vi "GFITS_getInfo.vi"(10 "ID":string, 11 "Database RefNum in":T1) -> (2 "INFO":string[][](array[string]))   [LabVIEW 2016]
uses:
  DBSHAND/private/vis/DatabaseHand_RefNum.ctl
  DBSHAND/private/vis/DatabaseHand_Element_Get(2DArr).vi
panel:
  out "Info received":string[][](table)=[["TIME", "", "time"], ["DATE", "", "data"], ["HRANGLE", "", "hr angle"], ["AZ", "", "az"], ["EI", "", "ei"], ["AIRMASS", "", "airmass"], ["DOME", "", "dome"], ["", "", ""], ["", "", ""]]
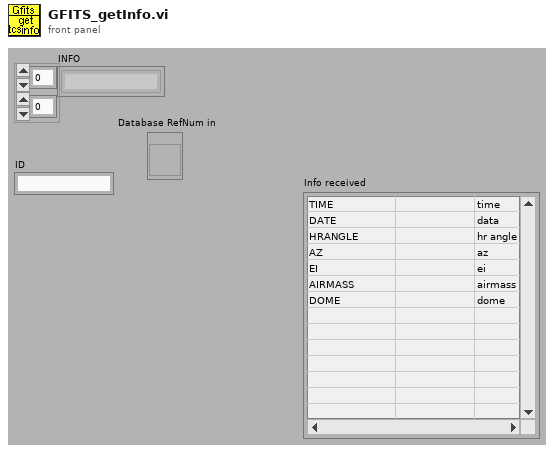
[diagram p1: front panel]
types:
  T1 = typedef "DatabaseHand_RefNum.ctl" = refnum<vi>
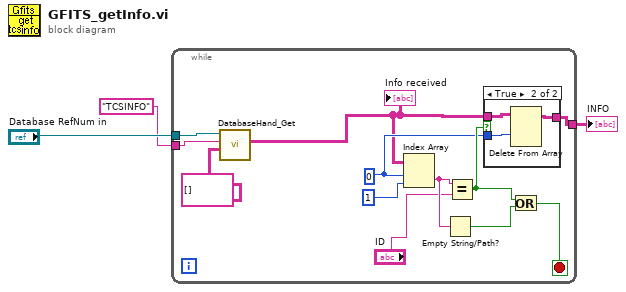
[diagram p0: block diagram]
diagram:
  n1 = while {
    tunnel: [w8] -> w3
    tunnel: "Database RefNum in" -> [w7]
    tunnel: "TCSINFO" ("name") -> [w6]
    stop <- w13 stop-if-true
    w10 = 0 ("Index (row)")
    n2 = call-poly "DatabaseHand_Get.vi"("default value"=string[][] [] ("INFO"), "name"=w6, "Database RefNum in"=w7) -> ("value"=w5:string[][])  [unwired: 2 in, 6 out]
    "Info received" <- w5
    n3 = Index Array(array=w5, index (row)=w10, index (col)=1 ("disabled index (col)")) -> (element=w15:string)
    n4 = Empty String/Path?(string/path=w15) -> (empty?=w14:bool)
    n5 = Equal?(x=w15, y="ID") -> (x = y?=w11:bool)
    n6 = case shown="True" w11 {
      tunnel: w5 -> [w16 w19]
      tunnel: w10 -> [_ w18]
      tunnel: [w16 w17] -> w8
      frame False {
      }
      frame True {
        n7 = Delete From Array(array=w19, index (row)=w18) -> (array with subset deleted=w17:string[][])  [unwired: 2 in, 1 out]
      }
    }
    n8 = Or(x=w11, y=w14) -> (x .or. y?=w13:bool)
  }
  "INFO" <- w3
